vi "Import_variable.vi"() -> ()   [LabVIEW 2018]
panel:
  out "Fullscale":i64
  out "Zero Offset":i16
  out "Calparam":i64[](array[numeric])
  out "Initial Tare":i64[](array[numeric])
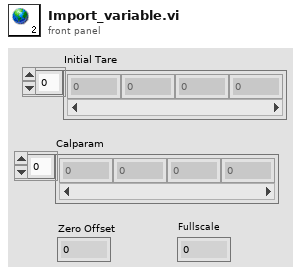
[diagram p1: front panel]
diagram:
